vi "Actor Core.vi"(8 "error In":errorcluster, 11 "Counter.lvclass":refnum<class "Counter.lvclass">) -> (0 "error out":errorcluster, 3 "Actor Output":refnum<class "Counter.lvclass">)   [LabVIEW 2018, in "Counter.lvclass"]
uses:
  Counter Class/Counter.lvclass
  Counter Class/Counter.lvclass/Counter.ctl
  Message Class/Message.lvclass
panel:
  out "Current Count":cdb
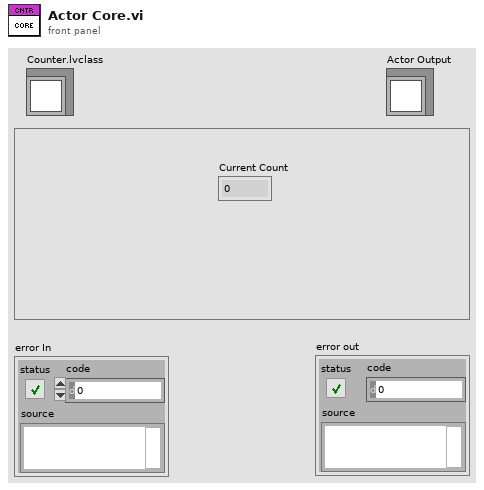
[diagram p1: front panel]
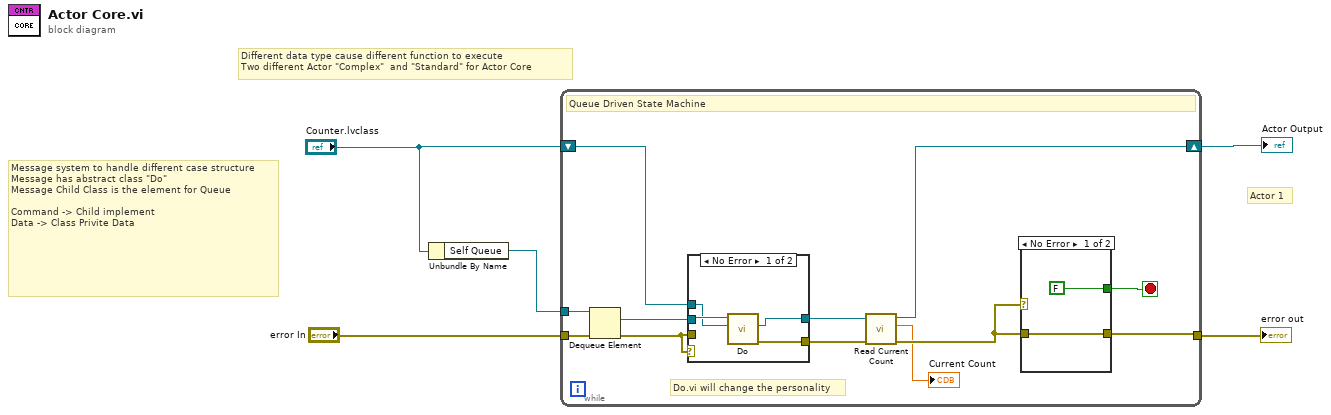
[diagram p0: block diagram]
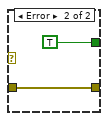
[diagram p2: hidden frame]
diagram:
  # "Actor 1"
  # "Message system to handle different case structure \nMessage has abstract class \"Do\"\nMessage Child Class is the element for Queue\n\nCommand -> Child implement \nData -> Class Privite Data"
  # "Different data type cause different function to execute \nTwo different Actor \"Complex\"  and \"Standard\" for Actor Core"
  n1 = Unbundle By Name("Counter.lvclass") -> ("Self Queue"=w3:refnum<queue>)
  n2 = while {
    tunnel: w3 -> [w16]
    shift-right: [w8] -> w5
    shift-left: "Counter.lvclass" -> [w6]
    tunnel: "error In" -> [w17]
    tunnel: [w13] -> w4
    stop <- w12 stop-if-true
    # "Do.vi will change the personality"
    # "Queue Driven State Machine"
    n3 = Dequeue Element(queue=w16, error in (no error)=w17) -> (element=w15:refnum<class "Message.lvclass">, error out=w14:errorcluster)  [unwired: 1 in, 2 out]
    n4 = case shown="No Error" w14 {
      tunnel: w15 -> [w25 _]
      tunnel: w6 -> [w24 w26]
      tunnel: [w23 w26] -> w11
      tunnel: [w22 w27] -> w10
      tunnel: w14 -> [_ w27]
      frame No Error {
        n5 = call-dynamic "Do.vi"("Counter In"=w24, "Message in"=w25) -> ("error out"=w22:errorcluster, "Counter Out"=w23:refnum<class "Counter.lvclass">)  [unwired: 7 in, 1 out]
      }
      frame Error {
      }
    }
    n6 = call-dynamic "Read Current Count.vi"("error in (no error)"=w10, "Counter in"=w11) -> ("error out"=w9:errorcluster, "Current Count"=→"Current Count":cdb, "Counter out"=w8:refnum<class "Counter.lvclass">)  [unwired: 7 in]
    n7 = case shown="No Error" w9 {
      tunnel: w9 -> [w19 w21]
      tunnel: [w19 w21] -> w13
      tunnel: [FALSE TRUE] -> w12
      frame No Error {
      }
      frame Error {
      }
    }
  }
  "Actor Output" <- w5
  "error out" <- w4
